vi "doAction.vi"(8 "error in (no error)":errorcluster, 10 "ContextData":refnum<class "ContextData.lvclass">, 11 "Run in":refnum<class "User State 1.lvclass">) -> (0 "error out":errorcluster, 2 "ContextData Out":refnum<class "ContextData.lvclass">, 3 "Run out":refnum<class "User State 1.lvclass">)   [LabVIEW 2019, in "User State 1.lvclass"]
uses:
  User State 1.lvclass
  ContextData/ContextData.lvclass
  ContextData/ContextData.lvclass/ContextData.ctl
  State/State.lvclass
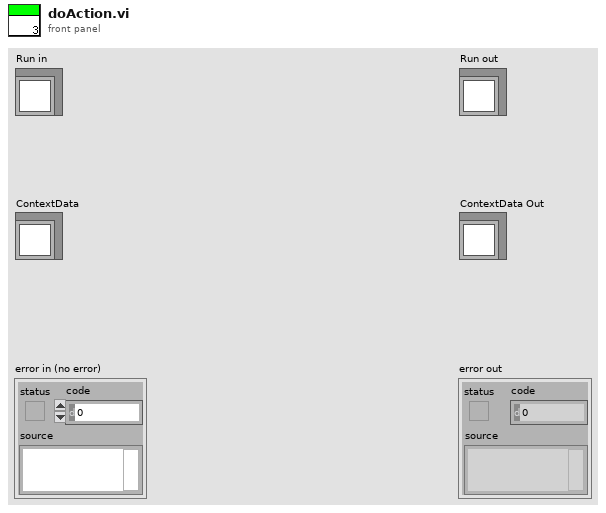
[diagram p1: front panel]
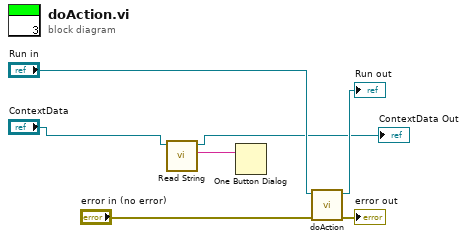
[diagram p0: block diagram]
diagram:
  n1 = call "Read String.vi"("ContextData in"="ContextData") -> ("String <Replace Me>"=w3:string, "ContextData out"=→"ContextData Out":refnum<class "ContextData.lvclass">)  [unwired: 8 in, 1 out]
  n2 = One Button Dialog(message=w3) -> ()  [unwired: 1 in, 1 out]
  n3 = call-parent "doAction.vi"("error in (no error)"="error in (no error)", "State in"="Run in") -> ("error out"=→"error out":errorcluster, "State out"=→"Run out":refnum<class "User State 1.lvclass">)  [unwired: 7 in, 1 out]
